vi "End Battle.vi"   [LabVIEW 2015, in "SB SubVIs.lvlib"]
uses:
  SB SubVIs.lvlib
  Square/Square.lvclass
  Square/Square.lvclass/Square.ctl
  Square/Read Name.vi
  Square/Read Victory Speech.vi
  Globals.vi
types:
  T1 = typedef "SB Type Defs.lvlib/UI Refs.ctl" = cluster{"Battlefield":refnum<vi>, "Dashboard":refnum<vi>, "End Battle":refnum<vi>, "Time Limit":refnum<vi>}
  T2 = typedef "SB Type Defs.lvlib/Dashboard.ctl" = cluster{"Color":u32, "Player":i32, "Status":string, "Add Player":T3}
  T3 = typedef "SB Type Defs.lvlib/Player Added.ctl" = bool
  T4 = typedef "SB Type Defs.lvlib/Square Cluster.ctl" = cluster{"Attacked?":bool, "DVR":refnum<data-value>, "Team":i32, "Player":i32, "Next Turn":i32, "Penalty":i32}
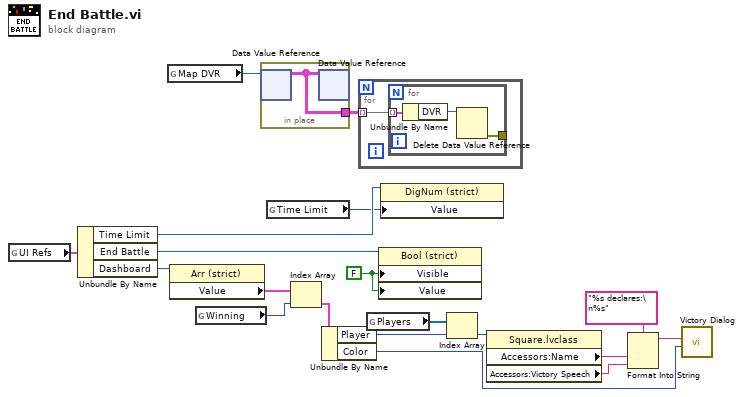
[diagram p0: block diagram]
diagram:
  w10 = FALSE ("Visible")
  n1 = global read "Globals.vi" "UI Refs"() -> (w12:T1)
  n2 = Unbundle By Name(w12) -> ("Time Limit"=w8:refnum<vi>, "End Battle"=w11:refnum<vi>, "Dashboard"=w6:refnum<vi>)
  n3 = global read "Globals.vi" "Map DVR"() -> (w13:refnum<data-value>)
  n4 = property class="Arr (strict)"(reference=w6) -> ("Value"=w5:T2[])  [unwired: 1 in, 2 out]
  n5 = global read "Globals.vi" "Winning"() -> (w4:i32)
  n6 = in-place {
    in-place-border: [w20] -> w19
    n7 = in-place-dvr #1(w13) -> (w20:T4[][])  [unwired: 1 out]
    n8 = in-place-dvr #1(w20) -> ()  [unwired: 2 out]
  }
  n9 = global read "Globals.vi" "Time Limit"() -> (w7:i32)
  n10 = Index Array(array=w5, index=w4) -> (element=w3:T2)
  n11 = Unbundle By Name(w3) -> ("Player"=w2:i32, "Color"=w1:u32)
  n12 = for {
    tunnel: w19 -> [w21] mode=indexing
    n13 = for {
      tunnel: w21 -> [w23] mode=indexing
      tunnel: [w22] -> _
      n14 = Unbundle By Name(w23) -> ("DVR"=w24:refnum<data-value>)
      n15 = Delete Data Value Reference(data value reference=w24) -> (error out=w22:errorcluster)  [unwired: 1 in, 1 out]
    }
  }
  n16 = global read "Globals.vi" "Players"() -> (w9:refnum<class "Square.lvclass">[])
  n17 = property on="Property Node" class="Bool (strict)"(reference=w11, "Visible"=w10, "Value"=w10) -> ()  [unwired: 1 in, 2 out]
  n18 = property class="DigNum (strict)"(reference=w8, "Value"=w7) -> ()  [unwired: 1 in, 2 out]
  n19 = Index Array(array=w9, index=w2) -> (element=w16:refnum<class "Square.lvclass">)
  n20 = property class="Square.lvclass"(reference=w16) -> ("Accessors:Name"=w15:string, "Accessors:Victory Speech"=w14:string)  [unwired: 1 in, 2 out]
  n21 = Format Into String(format string="%s declares:\n%s", w15, w14) -> (resulting string=w18:string)  [unwired: 2 in, 1 out]
  n22 = call "Victory Dialog.vi"("Pane Color"=w1, "Victory Phrase"=w18) -> ()  [unwired: 10 in]
